vi "TestExec.Health, Set Error.vi"(7 "Module Q Name":string, 8 "error in":errorcluster, 10 "Error":errorcluster, 11 "Q In":refnum<queue>) -> (0 "error out":errorcluster)   [LabVIEW 2018]
uses:
  <vilib>/KATE/Queues/Q.Element.ctl
  TestExec.Health State Command.ctl
  <vilib>/KATE/Queues/Queue Utils.lvlib
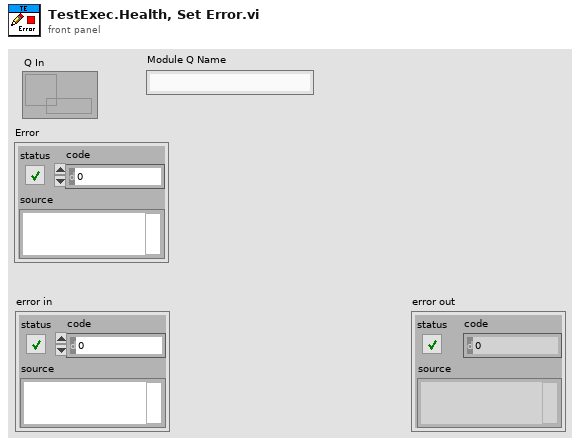
[diagram p1: front panel]
types:
  T1 = typedef "TestExec.Health State Command.ctl" = enum16{"Update", "Clear All", "Clear Warnings", "Clear Errors", "Set Warning", "Set Error"}
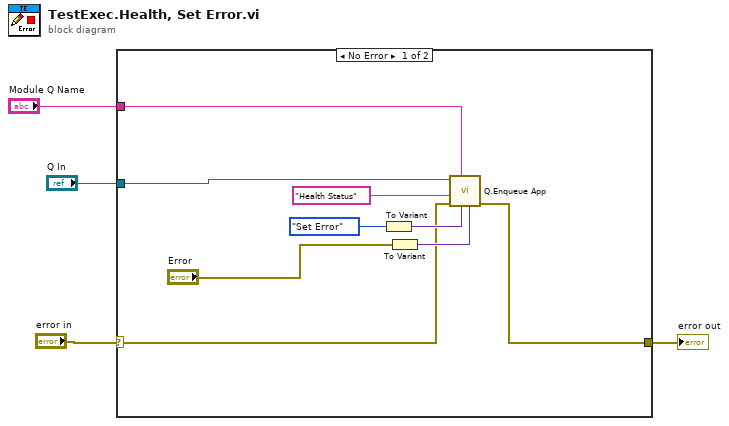
[diagram p0: block diagram]
diagram:
  n1 = case shown="No Error" "error in" {
    selector: "error in" -> [w8 w14]
    tunnel: [w9 w14] -> w3
    tunnel: "Q In" -> [w5 _]
    tunnel: "Module Q Name" -> [w6 _]
    frame No Error {
      n2 = To Variant(anything=TestExec.Health_State_Command."Set Error" ("Health State Cmd")) -> (Variant=w12:variant)
      n3 = To Variant(anything="Error") -> (Variant=w13:variant)
      n4 = call <vilib>:"Q.Enqueue App.vi"("Data2"=w13, "Data1"=w12, "Q Name"=w6, "Error In"=w8, "Task Name"="Health Status", "Q In"=w5) -> ("error out"=w9:errorcluster)  [unwired: 4 in, 1 out]
    }
    frame Error {
    }
  }
  "error out" <- w3
